vi "type_20_string_three_segments.vi"   [LabVIEW 2010]
types:
  T1 = enum16{"open", "open or create", "create or replace", "create", "open (read-only)"}
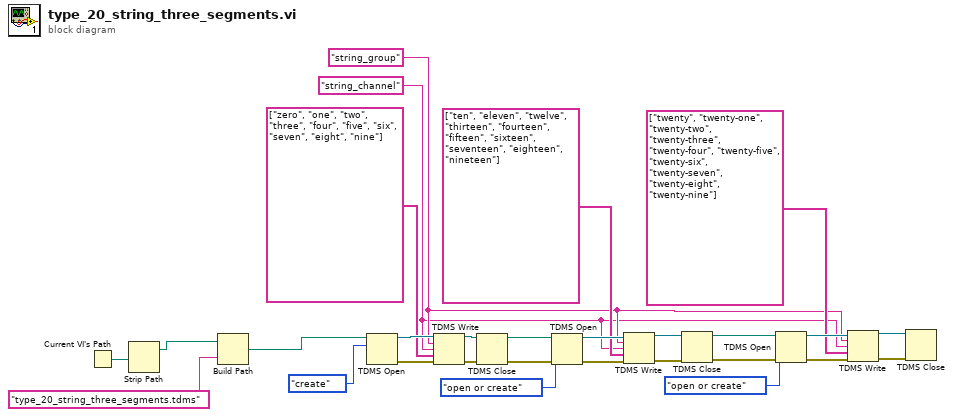
[diagram p0: block diagram]
diagram:
  w1 = "string_channel" ("channel name(s) in (Untitled)")
  w2 = "string_group" ("group name in (Untitled)")
  n1 = Current VI's Path() -> (path=w22:path)
  n2 = Strip Path(path=w22) -> (stripped path=w21:path)  [unwired: 1 out]
  n3 = Build Path(base path=w21, name or relative path="type_20_string_three_segments.tdms") -> (appended path=w19:path)
  n4 = TDMS Open(10:T1."create" ("operation (0:open)"), 11:w19) -> (0:w28:errorcluster, 3:w27:refnum<k34>)  [unwired: 4 in]
  n5 = TDMS Write(0:w27, 5:w2, 7:w1, 9:string[] ["zero", "one", "two", "three", "four", "five", "six", "seven", "eight", "nine"] ("channel name(s) in (Untitled)"), 11:w28) -> (4:w24:refnum<k34>, 15:w23:errorcluster)  [unwired: 1 in, 2 out]
  n6 = TDMS Close(8:w23, 11:w24) -> (0:w16:errorcluster, 3:w18:path)
  n7 = TDMS Open(8:w16, 10:T1."open or create" ("operation (0:open)"), 11:w18) -> (0:w15:errorcluster, 3:w14:refnum<k34>)  [unwired: 3 in]
  n8 = TDMS Write(0:w14, 5:w2, 7:w1, 9:string[] ["ten", "eleven", "twelve", "thirteen", "fourteen", "fifteen", "sixteen", "seventeen", "eighteen", "nineteen"] ("channel name(s) in (Untitled)"), 11:w15) -> (4:w11:refnum<k34>, 15:w12:errorcluster)  [unwired: 1 in, 2 out]
  n9 = TDMS Close(8:w12, 11:w11) -> (0:w4:errorcluster, 3:w5:path)
  n10 = TDMS Open(8:w4, 10:T1."open or create" ("operation (0:open)"), 11:w5) -> (0:w9:errorcluster, 3:w8:refnum<k34>)  [unwired: 3 in]
  n11 = TDMS Write(0:w8, 5:w2, 7:w1, 9:string[] ["twenty", "twenty-one", "twenty-two", "twenty-three", "twenty-four", "twenty-five", "twenty-six", "twenty-seven", "twenty-eight", "twenty-nine"] ("channel name(s) in (Untitled)"), 11:w9) -> (4:w6:refnum<k34>, 15:w7:errorcluster)  [unwired: 1 in, 2 out]
  n12 = TDMS Close(8:w7, 11:w6) -> ()  [unwired: 2 out]
